vi "custom_code_example.vi"() -> ()   [LabVIEW 2016]
uses:
  federate_library/objects_and_interfaces/InteractionRoot.C2WInteractionRoot.TMYWeather.ctl
  utilities/runtime/support/controls/hla_messaging_coordinator_actions.ctl
  utilities/runtime/support/controls/messaging_processor_params.ctl
  federate_library/objects_and_interfaces/ObjectRoot.Setpoint.ctl
  utilities/runtime/support/controls/event_assistant_actions.ctl
  utilities/runtime/support/controls/user_event_item.ctl
  utilities/runtime/support/controls/user_events.ctl
  federate_library/hla_queues/instances/hla_outgoing_queue_instance_2.vi
  federate_library/hla_queues/instances/hla_incoming_queue_instance_10.vi
  federate_library/hla_queues/instances/hla_incoming_queue_instance_1.vi
  federate_library/hla_queues/instances/hla_incoming_queue_instance_4.vi
panel:
  out "%_1":dbl
  out "%_2":dbl
  in  "stop":bool
  in  "tdelay":u32(knob) scale=0.0..10.0
  out "timestep":dbl
  in  "sp_2_down":bool
  in  "sp_2_up":bool
  out "iat_2":dbl
  out "sp_2":dbl
  in  "sp_1_down":bool
  in  "sp_1_up":bool
  out "iat_1":dbl
  out "sp_1":dbl
  out "weather (in)":T1[](array[typedef])
  in  "error in (no error)":errorcluster
  out "error out":errorcluster
  # "ZONE 1"
  # "ZONE 2"
  # "IAT"
  # "IAT"
  # "time delay (s)"
  # "```"
  # "%"
  # "%"
  # "SETPOINT"
  # "SETPOINT"
  # "% open"
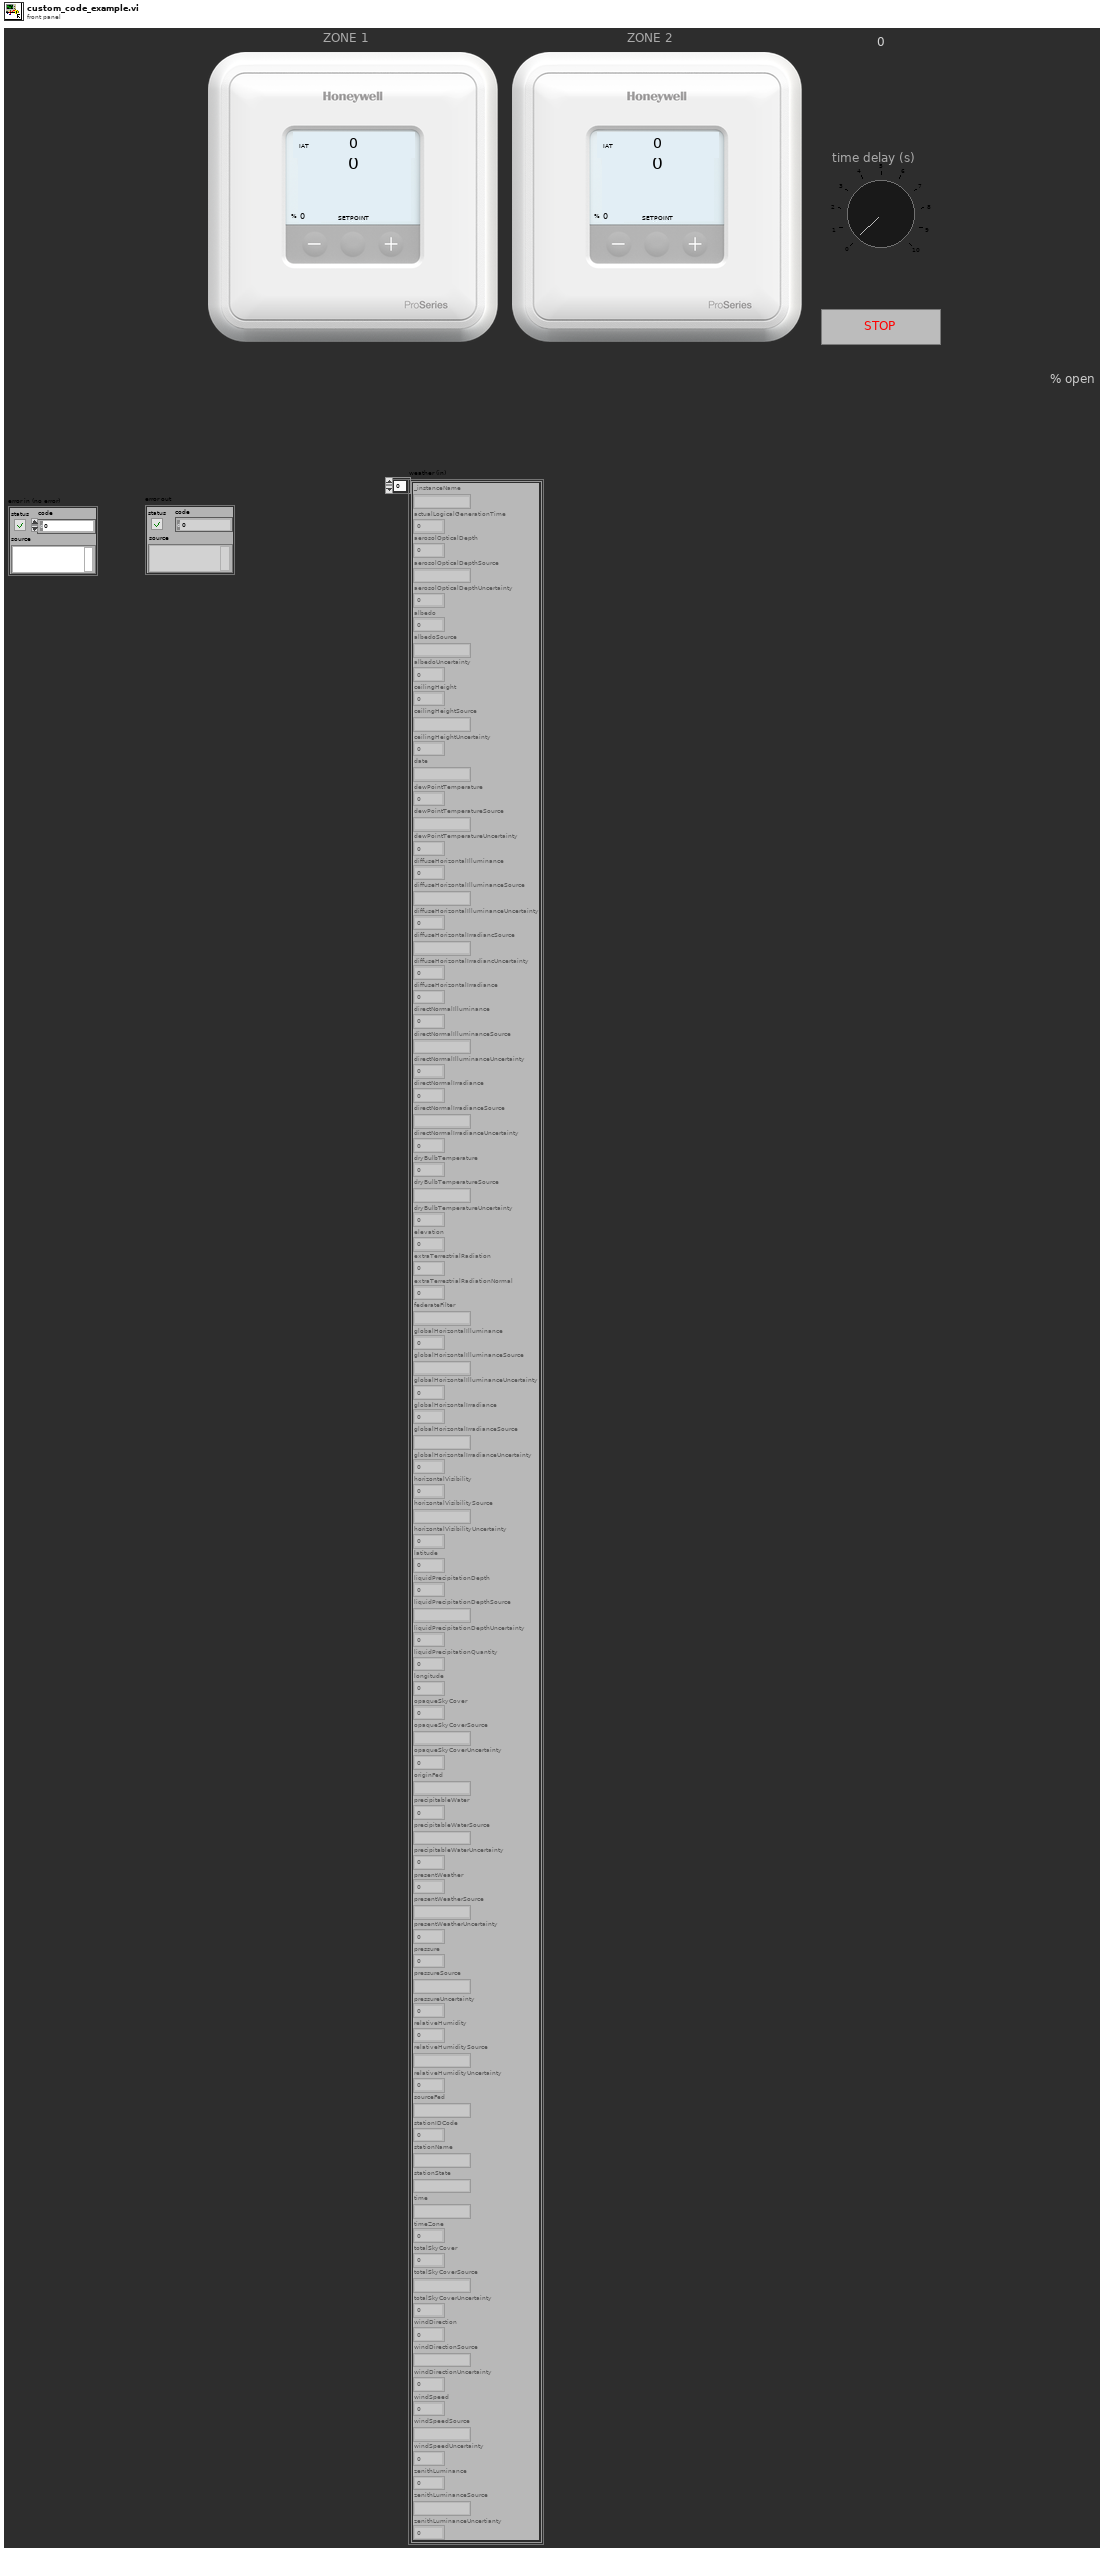
[diagram p1: front panel]
types:
  T1 = typedef "InteractionRoot.C2WInteractionRoot.TMYWeather.ctl" = cluster{"_instanceName":string, "actualLogicalGenerationTime":dbl, "aerosolOpticalDepth":dbl, "aerosolOpticalDepthSource":string, "aerosolOpticalDepthUncertainty":dbl, "albedo":dbl, "albedoSource":string, "albedoUncertainty":dbl, "ceilingHeight":dbl, "ceilingHeightSource":string, "ceilingHeightUncertainty":dbl, "date":string, "dewPointTemperature":dbl, "dewPointTemperatureSource":string, "dewPointTemperatureUncertainty":dbl, "diffuseHorizontalIlluminance":dbl, "diffuseHorizontalIlluminanceSource":string, "diffuseHorizontalIlluminanceUncertainty":dbl, "diffuseHorizontalIrradiancSource":string, "diffuseHorizontalIrradiancUncertainty":dbl, "diffuseHorizontalIrradiance":dbl, "directNormalIlluminance":dbl, "directNormalIlluminanceSource":string, "directNormalIlluminanceUncertainty":dbl, "directNormalIrradiance":dbl, "directNormalIrradianceSource":string, "directNormalIrradianceUncertainty":dbl, "dryBulbTemperature":dbl, "dryBulbTemperatureSource":string, "dryBulbTemperatureUncertainty":dbl, "elevation":dbl, "extraTerrestrialRadiation":dbl, "extraTerrestrialRadiationNormal":dbl, "federateFilter":string, "globalHorizontalIlluminance":dbl, "globalHorizontalIlluminanceSource":string, "globalHorizontalIlluminanceUncertainty":dbl, "globalHorizontalIrradiance":dbl, "globalHorizontalIrradianceSource":string, "globalHorizontalIrradianceUncertainty":dbl, "horizontalVisibility":dbl, "horizontalVisibilitySource":string, "horizontalVisibilityUncertainty":dbl, "latitude":dbl, "liquidPrecipitationDepth":dbl, "liquidPrecipitationDepthSource":string, "liquidPrecipitationDepthUncertainty":dbl, "liquidPrecipitationQuantity":dbl, "longitude":dbl, "opaqueSkyCover":dbl, "opaqueSkyCoverSource":string, "opaqueSkyCoverUncertainty":dbl, "originFed":string, "precipitableWater":dbl, "precipitableWaterSource":string, "precipitableWaterUncertainty":dbl, "presentWeather":dbl, "presentWeatherSource":string, "presentWeatherUncertainty":dbl, "pressure":dbl, "pressureSource":string, "pressureUncertainty":dbl, "relativeHumidity":dbl, "relativeHumiditySource":string, "relativeHumidityUncertainty":dbl, "sourceFed":string, "stationIDCode":i32, "stationName":string, "stationState":string, "time":string, "timeZone":dbl, "totalSkyCover":dbl, "totalSkyCoverSource":string, "totalSkyCoverUncertainty":dbl, "windDirection":dbl, "windDirectionSource":string, "windDirectionUncertainty":dbl, "windSpeed":dbl, "windSpeedSource":string, "windSpeedUncertainty":dbl, "zenithLuminance":dbl, "zenithLuminanceSource":string, "zenithLuminanceUncertianty":dbl}
  T2 = typedef "hla_messaging_coordinator_actions.ctl" = enum16{"activate", "get_event_ref", "terminate"}
  T3 = typedef "messaging_processor_params.ctl" = cluster{"hla_adapter_port":u16, "hla_adapter_ip":string, "listener_port":u16}
  T4 = typedef "ObjectRoot.Setpoint.ctl" = cluster{"_instanceName":string, "Occupied":bool, "ZoneTempSP":dbl, "ZoneName":string}
  T5 = typedef "ObjectRoot.ZoneState.ctl" = cluster{"_instanceName":string, "CoolingOverride":bool, "IATemperature":dbl, "PowerTotal":dbl, "ZoneName":string}
  T6 = typedef "ObjectRoot.ControllerState.ctl" = cluster{"_instanceName":string, "DamperPostionPct":i32, "ZoneName":string}
  T7 = typedef "user_event_item.ctl" = cluster{"event":T8, "data":variant}
  T8 = typedef "user_events.ctl" = enum16{"abort", "do-step", "sim-end"}
  T9 = typedef "event_assistant_actions.ctl" = enum16{"--- unused ---", "destroy", "fire", "get_ref", "init"}
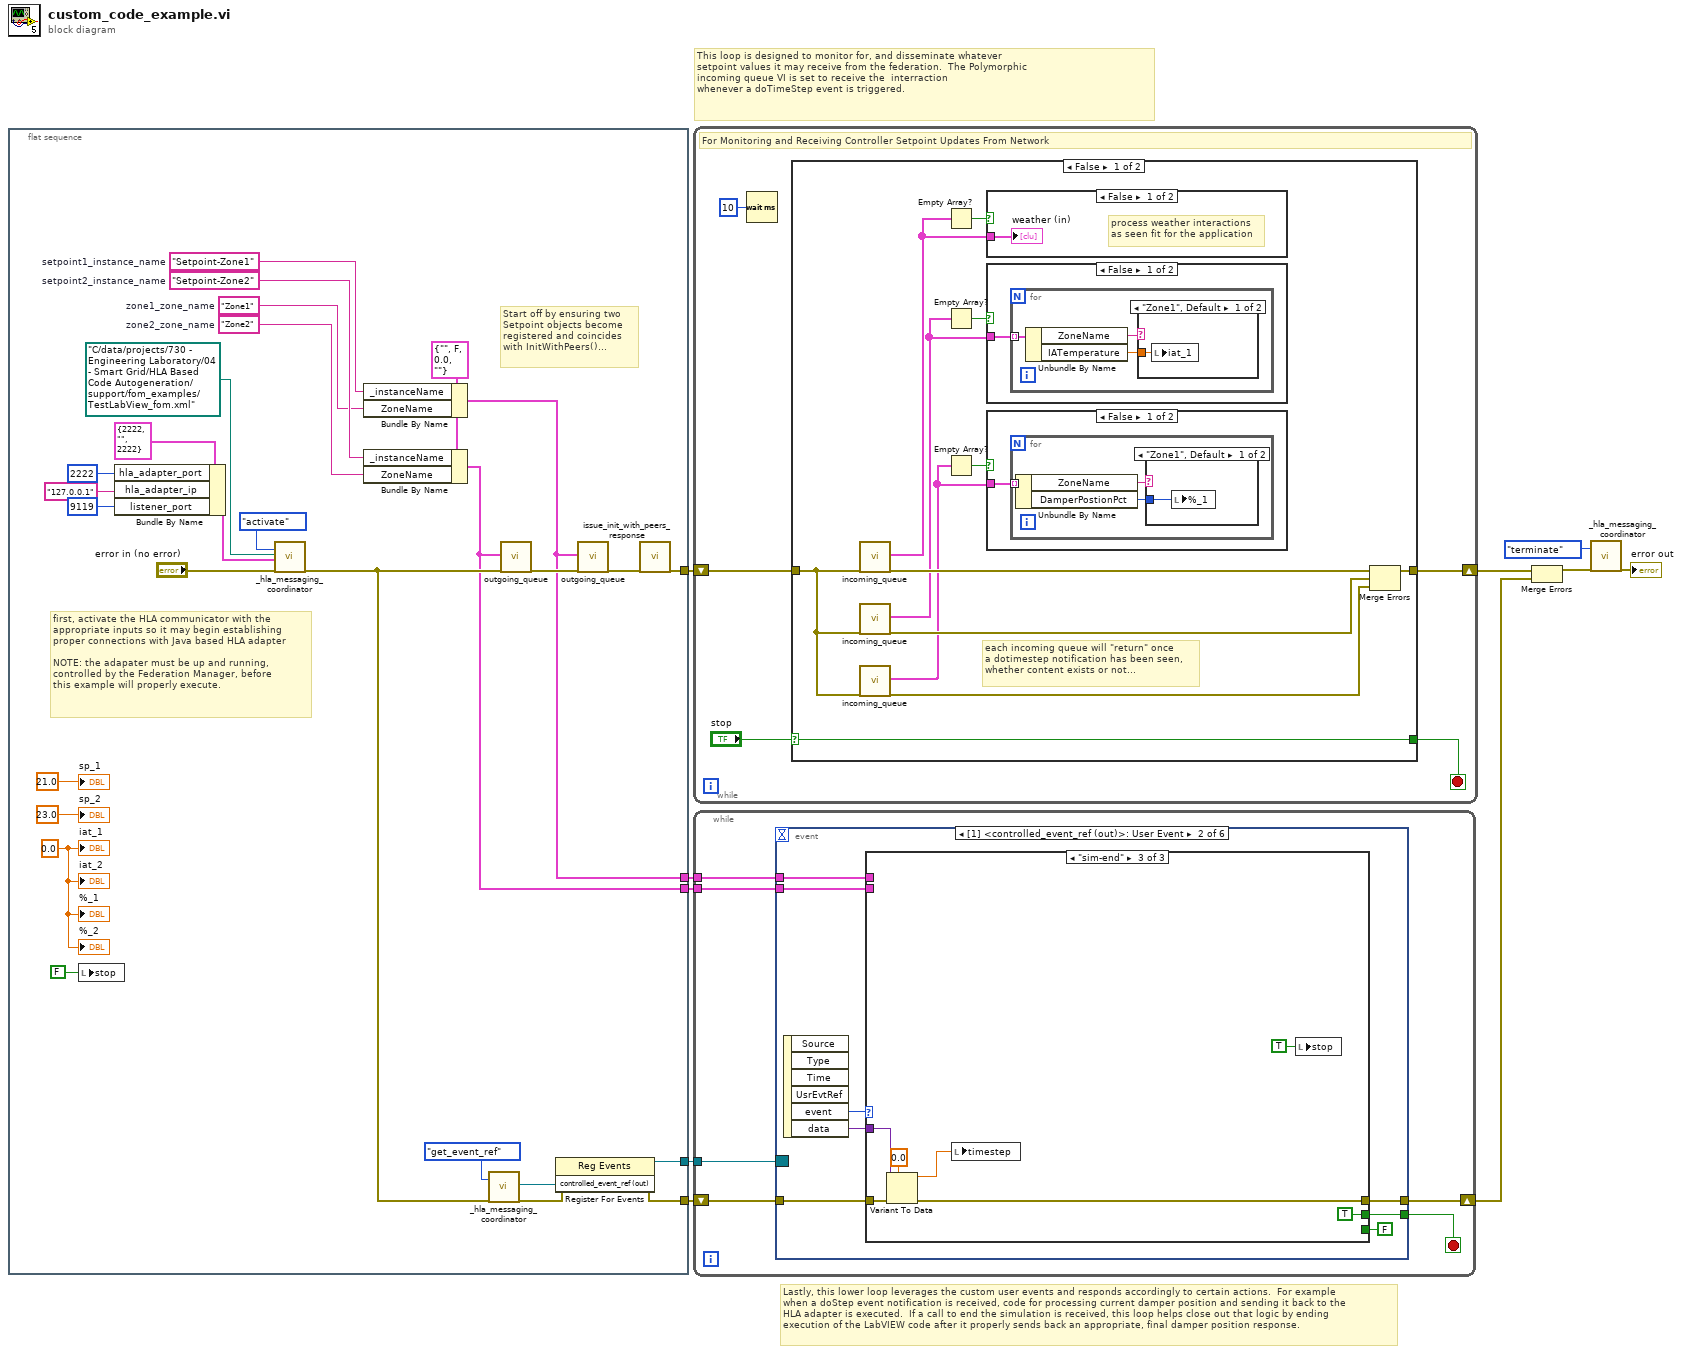
[diagram p0: block diagram]
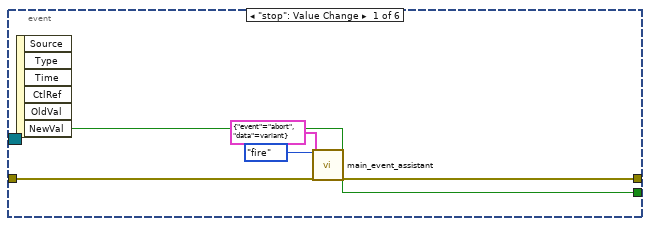
[diagram p2: hidden frame]
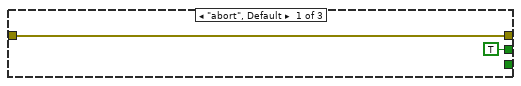
[diagram p3: hidden frame]
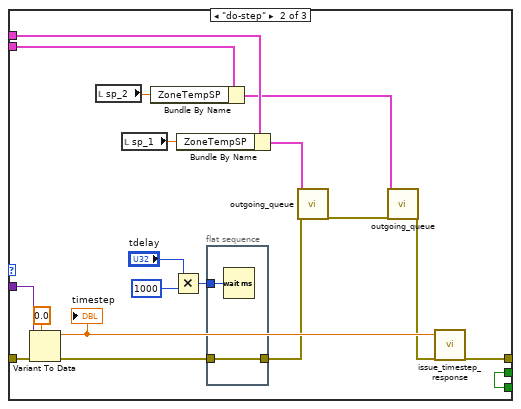
[diagram p4: hidden frame]
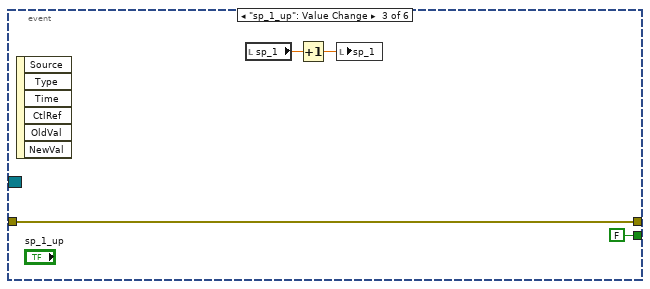
[diagram p5: hidden frame]
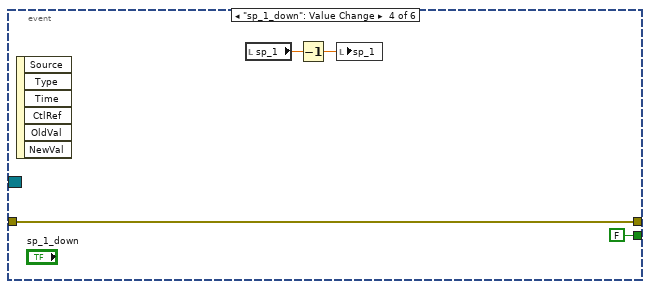
[diagram p6: hidden frame]
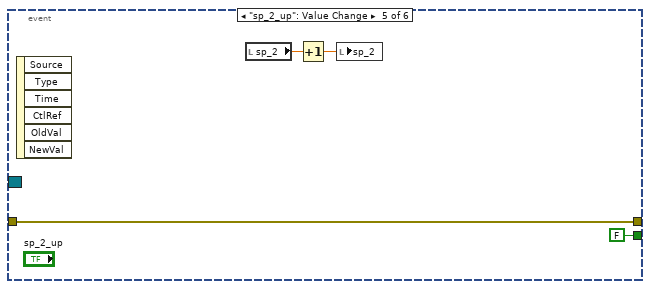
[diagram p7: hidden frame]
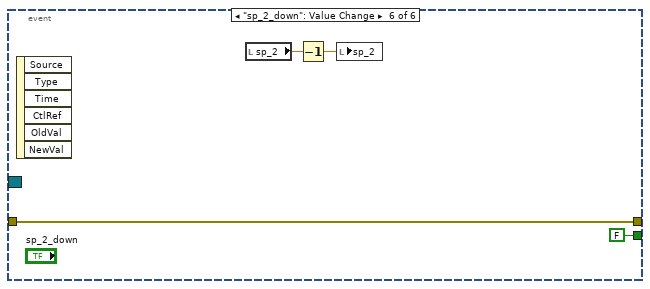
[diagram p8: hidden frame]
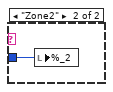
[diagram p9: hidden frame]
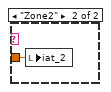
[diagram p11: hidden frame]
diagram:
  # "This loop is designed to monitor for, and disseminate whatever\nsetpoint values it may receive from the federation.  The Polymorphic\nincoming queue VI is set to receive the  interraction\nwhenever a doTimeStep event is triggered."
  # "Lastly, this lower loop leverages the custom user events and responds accordingly to certain actions.  For example\nwhen a doStep event notification is received, code for processing current damper position and sending it back to the\nHLA adapter is executed.  If a call to end the simulation is received, this loop helps close out that logic by ending\nexecution of the LabVIEW code after it properly sends back an appropriate, final damper position response."
  n1 = flat-sequence {
    tunnel: [w19] -> w8
    tunnel: [w34] -> w7
    tunnel: [w33] -> w3
    tunnel: [w18] -> w2
    tunnel: [w17] -> w1
    frame #0 {
      w12 = "Zone2"  # zone2_zone_name
      w14 = "Setpoint-Zone2"  # setpoint2_instance_name
      w13 = "Zone1"  # zone1_zone_name
      w11 = 0.0 ("iat_1")
      w21 = "Setpoint-Zone1"  # setpoint1_instance_name
      w22 = T4 {"_instanceName"="", "Occupied"=FALSE, "ZoneTempSP"=0.0, "ZoneName"=""} ("ObjectRoot.Setpoint")
      # "Start off by ensuring two\nSetpoint objects become \nregistered and coincides\nwith InitWithPeers()..."
      # "first, activate the HLA communicator with the\nappropriate inputs so it may begin establishing\nproper connections with Java based HLA adapter\n\nNOTE: the adapater must be up and running, \ncontrolled by the Federation Manager, before\nthis example will properly execute."
      n2 = local write "stop"(FALSE ("stop")) -> ()
      n3 = Bundle By Name(cluster=T3 {"hla_adapter_port"=2222, "hla_adapter_ip"="", "listener_port"=2222} ("params"), "hla_adapter_port"=u16 2222 ("remote port or service name"), "hla_adapter_ip"="127.0.0.1" ("address"), "listener_port"=u16 9119 ("remote port or service name")) -> (w28:T3)
      n4 = call "_hla_messaging_coordinator.vi"("actions"=hla_messaging_coordinator_actions."activate", "fom_path (in)"=path "C:/data/projects/730 - Engineering Laboratory/04 - Smart Grid/HLA Based Code Autogeneration/support/fom_examples/TestLabView_fom.xml", "params"=w28, "error in (no error)"="error in (no error)") -> ("error out"=w24:errorcluster)  [unwired: 14 in, 1 out]
      n5 = Bundle By Name(cluster=w22, "_instanceName"=w21, "ZoneName"=w13) -> (w18:T4)
      n6 = Bundle By Name(cluster=w22, "_instanceName"=w14, "ZoneName"=w12) -> (w17:T4)
      n7 = call "_hla_messaging_coordinator.vi"("actions"=hla_messaging_coordinator_actions."get_event_ref", "error in (no error)"=w24) -> ("controlled_event_ref (out)"=w25:refnum<user-event>, "error out"=w26:errorcluster)  [unwired: 16 in]
      n8 = call-poly "outgoing_queue.vi"("ObjectRoot.Setpoint"=w17, "error in (no error)"=w24) -> ("error out"=w23:errorcluster)  [unwired: 17 in]
      n9 = register-events(error in=w26, w25) -> (reference out=w33:refnum<event-registration>, error out=w34:errorcluster)  [unwired: 1 in]
      n10 = call-poly "outgoing_queue.vi"("ObjectRoot.Setpoint"=w18, "error in (no error)"=w23) -> ("error out"=w20:errorcluster)  [unwired: 17 in]
      n11 = call "issue_init_with_peers_response.vi"("error in (no error)"=w20) -> ("error out"=w19:errorcluster)  [unwired: 18 in]
      "sp_1" <- 21.0 ("iat_1")
      "sp_2" <- 23.0 ("iat_1")
      "iat_2" <- w11
      "iat_1" <- w11
      "%_1" <- w11
      "%_2" <- w11
    }
  }
  n12 = while {
    shift-right: [w43] -> w6
    shift-left: w8 -> [w42]
    stop <- w40 stop-if-true
    # "For Monitoring and Receiving Controller Setpoint Updates From Network"
    n13 = Wait (ms)(milliseconds to wait=u32 10) -> ()  [unwired: 1 out]
    n14 = case shown="False" "stop" {
      selector: "stop" -> [w44 w69]
      tunnel: [w53 w70] -> w43
      tunnel: w42 -> [w52 w70]
      tunnel: [w44 w69] -> w40
      frame False {
        # "each incoming queue will \"return\" once\na dotimestep notification has been seen,\nwhether content exists or not..."
        n15 = call-poly "incoming_queue.vi"("error in (no error)"=w52) -> ("entity_array"=w49:T1[], "error out"=w55:errorcluster)  [unwired: 15 in, 2 out]
        n16 = call-poly "incoming_queue.vi"("error in (no error)"=w52) -> ("entity_array"=w47:T5[], "error out"=w54:errorcluster)  [unwired: 15 in, 2 out]
        n17 = call-poly "incoming_queue.vi"("error in (no error)"=w52) -> ("entity_array"=w45:T6[], "error out"=w51:errorcluster)  [unwired: 15 in, 2 out]
        n18 = Empty Array?(array=w49) -> (empty?=w50:bool)
        n19 = Empty Array?(array=w47) -> (empty?=w48:bool)
        n20 = Empty Array?(array=w45) -> (empty?=w46:bool)
        n21 = case shown="False" w50 {
          tunnel: w49 -> [w68 _]
          frame False {
            # "process weather interactions\nas seen fit for the application"
            "weather (in)" <- w68
          }
          frame True {
          }
        }
        n22 = case shown="False" w48 {
          tunnel: w47 -> [w62 _]
          frame False {
            n23 = for {
              tunnel: w62 -> [w65] mode=indexing
              n24 = Unbundle By Name(w65) -> ("ZoneName"=w64:string, "IATemperature"=w63:dbl)
              n25 = case shown="\"Zone1\", Default" w64 {
                tunnel: w63 -> [w66 w67]
                frame "Zone1", Default {
                  n26 = local write "iat_1"(w66) -> ()
                }
                frame "Zone2" {
                  n27 = local write "iat_2"(w67) -> ()
                }
              }
            }
          }
          frame True {
          }
        }
        n28 = case shown="False" w46 {
          tunnel: w45 -> [w56 _]
          frame False {
            n29 = for {
              tunnel: w56 -> [w59] mode=indexing
              n30 = Unbundle By Name(w59) -> ("ZoneName"=w58:string, "DamperPostionPct"=w57:i32)
              n31 = case shown="\"Zone1\", Default" w58 {
                tunnel: w57 -> [w60 w61]
                frame "Zone1", Default {
                  n32 = local write "%_1"(w60) -> ()
                }
                frame "Zone2" {
                  n33 = local write "%_2"(w61) -> ()
                }
              }
            }
          }
          frame True {
          }
        }
        n34 = Merge Errors(w55, w54, w51) -> (w53:errorcluster)
      }
      frame True {
      }
    }
  }
  n35 = while {
    shift-right: [w75] -> w5
    shift-left: w7 -> [w76]
    tunnel: w3 -> [w73]
    tunnel: w2 -> [w72]
    tunnel: w1 -> [w71]
    stop <- w74 stop-if-true
    n36 = event shown="[1] <controlled_event_ref (out)>: User Event" {
      selector: w73 -> [_ _ _ _ _ _]
      dyn-events: _ -> [_ _ _ _ _ _]
      timeout: _ -> [_ _ _ _ _ _]
      tunnel: w76 -> [w79 w89 w121 w125 w129 w133]
      tunnel: [w77 w84 w121 w125 w129 w133] -> w75
      tunnel: [w81 w86 FALSE ("NewVal") FALSE ("NewVal") FALSE ("NewVal") FALSE ("NewVal")] -> w74
      tunnel: w72 -> [_ w83 _ _ _ _]
      tunnel: w71 -> [_ w82 _ _ _ _]
      event "stop": Value Change {
        n37 = event-data() -> ("NewVal"=w81:bool)  [unwired: 1 in, 5 out]
        n38 = call "main_event_assistant.vi"("event_action (enq_behind = def)"=event_assistant_actions."fire", "event_item (in)"=T7 {"event"=enum."abort", "data"=variant}, "error in (no error)"=w79) -> ("error out"=w77:errorcluster)  [unwired: 15 in, 1 out]
      }
      event User Event {
        n39 = event-data() -> ("event"=w87:T8, "data"=w88:variant)  [unwired: 1 in, 4 out]
        n40 = case shown="\"sim-end\"" w87 {
          tunnel: w89 -> [w91 w110 w119]
          tunnel: [w91 w102 w113] -> w84
          tunnel: w88 -> [_ w109 w118]
          tunnel: [TRUE w107 TRUE] -> w86
          tunnel: FALSE -> [_ w107 _]
          tunnel: w83 -> [_ w98 _]
          tunnel: w82 -> [_ w95 _]
          frame "abort", Default {
          }
          frame "do-step" {
            n41 = Variant To Data(error in=w110, type=0.0, Variant=w109) -> (data=w101:dbl, error out=w103:errorcluster)
            "timestep" <- w101
            n42 = local read "sp_2"() -> (w92:dbl)
            n43 = local read "sp_1"() -> (w93:dbl)
            n44 = Bundle By Name(cluster=w95, "ZoneTempSP"=w92) -> (w94:T4)
            n45 = Multiply(x="tdelay", y=u32 1000) -> (x*y=w104:u32)
            n46 = Bundle By Name(cluster=w98, "ZoneTempSP"=w93) -> (w100:T4)
            n47 = flat-sequence {
              tunnel: w104 -> [w112]
              tunnel: [w111] -> w99
              tunnel: w103 -> [w111]
              frame #0 {
                n48 = Wait (ms)(milliseconds to wait=w112) -> ()  [unwired: 1 out]
              }
            }
            n49 = call-poly "outgoing_queue.vi"("ObjectRoot.Setpoint"=w100, "error in (no error)"=w99) -> ("error out"=w97:errorcluster)  [unwired: 17 in]
            n50 = call-poly "outgoing_queue.vi"("ObjectRoot.Setpoint"=w94, "error in (no error)"=w97) -> ("error out"=w96:errorcluster)  [unwired: 17 in]
            n51 = call "issue_timestep_response.vi"("timestep (in)"=w101, "error in (no error)"=w96) -> ("error out"=w102:errorcluster)  [unwired: 17 in]
          }
          frame "sim-end" {
            n52 = Variant To Data(error in=w119, type=0.0, Variant=w118) -> (data=w116:dbl, error out=w113:errorcluster)
            n53 = local write "timestep"(w116) -> ()
            n54 = local write "stop"(TRUE ("stop")) -> ()
          }
        }
      }
      event "sp_1_up": Value Change {
        n55 = event-data() -> ()  [unwired: 1 in, 6 out]
        n56 = local read "sp_1"() -> (w122:dbl)
        n57 = Increment(x=w122) -> (x+1=w123:dbl)
        n58 = local write "sp_1"(w123) -> ()
      }
      event "sp_1_down": Value Change {
        n59 = event-data() -> ()  [unwired: 1 in, 6 out]
        n60 = local read "sp_1"() -> (w126:dbl)
        n61 = Decrement(x=w126) -> (x-1=w127:dbl)
        n62 = local write "sp_1"(w127) -> ()
      }
      event "sp_2_up": Value Change {
        n63 = event-data() -> ()  [unwired: 1 in, 6 out]
        n64 = local read "sp_2"() -> (w130:dbl)
        n65 = Increment(x=w130) -> (x+1=w131:dbl)
        n66 = local write "sp_2"(w131) -> ()
      }
      event "sp_2_down": Value Change {
        n67 = event-data() -> ()  [unwired: 1 in, 6 out]
        n68 = local read "sp_2"() -> (w134:dbl)
        n69 = Decrement(x=w134) -> (x-1=w135:dbl)
        n70 = local write "sp_2"(w135) -> ()
      }
    }
  }
  n71 = Merge Errors(w6, w5) -> (w4:errorcluster)
  n72 = call "_hla_messaging_coordinator.vi"("actions"=hla_messaging_coordinator_actions."terminate", "error in (no error)"=w4) -> ("error out"=→"error out":errorcluster)  [unwired: 16 in, 1 out]
